vi "While Loop Basics with Tunnels.vi"() -> ()   [LabVIEW 2020]
panel:
  out "Total Number of Iterations":i32
  in  "Stop":bool
  out "Current Iteration":i32
  out "Seconds":dbl
  out "Minutes":dbl
  out "Hours":dbl
  in  "Total Time in Seconds":dbl
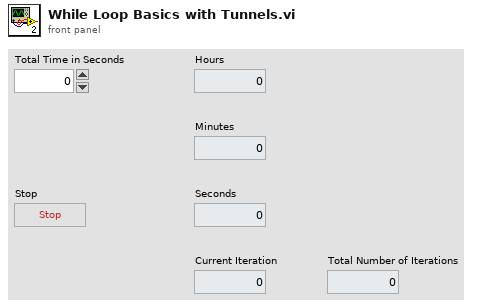
[diagram p1: front panel]
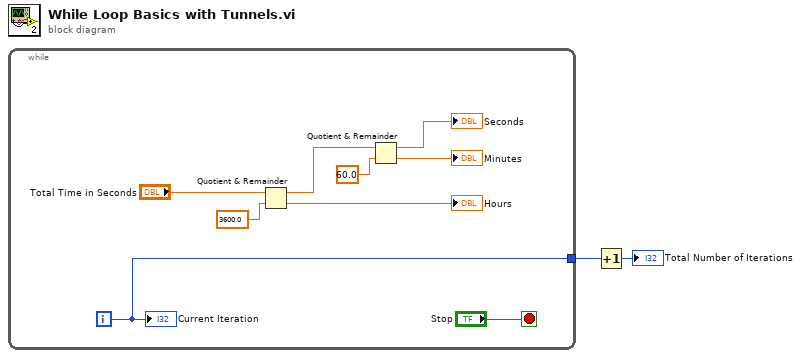
[diagram p0: block diagram]
diagram:
  n1 = while {
    tunnel: [w4] -> w2
    i -> [w4]
    stop <- "Stop" stop-if-true
    n2 = Quotient & Remainder(x="Total Time in Seconds", y=3600.0) -> (x-y*floor(x/y)=w9:dbl, floor(x/y)=→"Hours":dbl)
    n3 = Quotient & Remainder(x=w9, y=60.0) -> (x-y*floor(x/y)=→"Seconds":dbl, floor(x/y)=→"Minutes":dbl)
    "Current Iteration" <- w4
  }
  n4 = Increment(x=w2) -> (x+1=→"Total Number of Iterations":i32)
